vi "Main.vi"() -> ()   [LabVIEW 2018]
panel:
  out "error out":errorcluster
  in  "Button":bool
  in  "Stop":bool
  in  "Batch PDT FilePath":path
  in  "PDT *.csv FilePath":path=path "C:/Users/dev/Downloads/PDT.csv"
  out "String":string
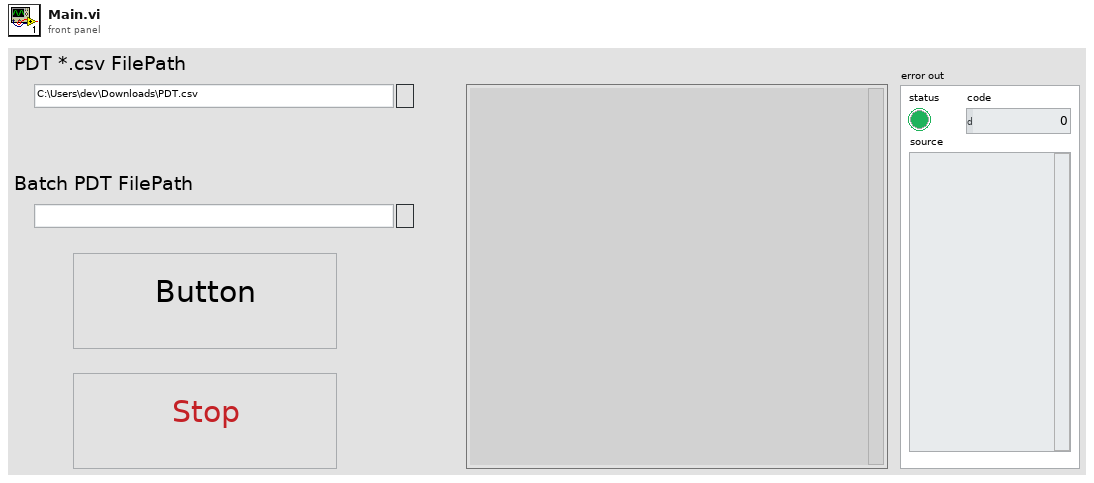
[diagram p1: front panel]
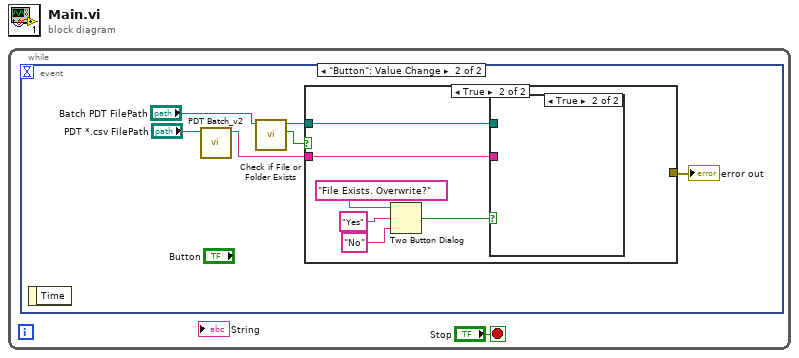
[diagram p0: block diagram]
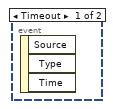
[diagram p2: hidden frame]
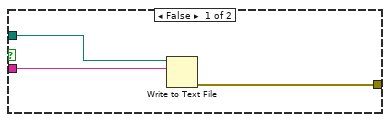
[diagram p3: hidden frame]
diagram:
  n1 = while {
    stop <- "Stop" stop-if-true
    n2 = event shown="[1] \"Button\": Value Change" {
      selector: _ -> [_ _]
      dyn-events: _ -> [_ _]
      timeout: _ -> [_ _]
      event Timeout {
        n3 = event-data() -> ()  [unwired: 1 in, 3 out]
      }
      event "Button": Value Change {
        n4 = event-data() -> ()  [unwired: 1 in, 1 out]
        n5 = call "PDT Batch_v2.vi"("PDT *.csv FilePath"="PDT *.csv FilePath") -> ("String"=w4:string)  [unwired: 10 in]
        n6 = call <vilib>:"Check if File or Folder Exists.vi"("path"="Batch PDT FilePath") -> ("file or folder exists?"=w5:bool, "dup path"=w3:path)  [unwired: 8 in, 1 out]
        n7 = case shown="True" w5 {
          tunnel: w4 -> [w10 w11]
          tunnel: w3 -> [w9 w12]
          tunnel: [w8 _] -> w2
          frame False {
            n8 = Write to Text File(file (use dialog)=w9, text=w10) -> (error out=w8:errorcluster)  [unwired: 2 in, 2 out]
          }
          frame True {
            n9 = Two Button Dialog(message="File Exists. Overwrite?", 1:"No" ("message"), 2:"Yes" ("message")) -> (T button?=w13:bool)
            n10 = case shown="True" w13 {
              tunnel: w12 -> [_ _]
              tunnel: w11 -> [_ _]
              frame False {
              }
              frame True {
              }
            }
          }
        }
        "error out" <- w2
      }
    }
  }
